vi "Generate Sine SweepV4.vi"() -> ()   [LabVIEW 2018]
uses:
  <vilib>/addons/_NISVFA/_Shared subVIs/Controls/svc_Channel Info.ctl
  <vilib>/addons/_NISVFA/_Shared subVIs/Controls/svc_Engineering Units Text Ring.ctl
  <vilib>/addons/_NISVFA/_Shared subVIs/Controls/svc_Weighting Filter Text Ring.ctl
  <vilib>/sound2/lvsound2.llb/Sound Output Task ID.ctl
  <vilib>/sound2/lvsound2.llb/Sound Input Task ID.ctl
  <vilib>/sound2/lvsound2.llb/Sound Data Format.ctl
  <vilib>/sound2/lvsound2.llb/Sampling Mode.ctl
  <vilib>/addons/Sound and Vibration/svt_Calibration/SVL Scale Voltage to EU (1 Ch).vi
  <vilib>/addons/_NISVFA/_Shared subVIs/Common/svc_Set SV Channel Info.vi
  <vilib>/addons/_NISVFA/_Shared subVIs/Common/svc_Set SV Channel Info (variant).vi
  <vilib>/addons/_NISVFA/_Shared subVIs/Common/SVL Set dB Reference (variant).vi
  <vilib>/sound2/lvsound2.llb/Sound Output Set Volume (Single).vi
  <vilib>/sound2/lvsound2.llb/Sound Output Write (DBL Single).vi
  <vilib>/sound2/lvsound2.llb/Sound Input Read (DBL).vi
  <vilib>/sound2/lvsound2.llb/Sound File Write Open.vi
  <vilib>/sound2/lvsound2.llb/Sound File Write (DBL Single).vi
  <vilib>/addons/_NISVFA/_Shared subVIs/Common/svc_Engineering Units to Unit Label.vi
  <vilib>/addons/_NISVFA/_Shared subVIs/Common/svc_Compute Scale Factor to Convert V to EU.vi
  <vilib>/addons/_NISVFA/_Shared subVIs/Common/svc_Compute Scale Factor to Convert C to EU.vi
  <vilib>/addons/_NISVFA/_Shared subVIs/Common/svc_Set dB ref if Pascal.vi
  <vilib>/addons/_NISVFA/_Shared subVIs/Common/svc_Caller VI Returned in Error Source.vi
  <vilib>/measure/maspectr.llb/FFT Spectrum (Mag-Phase) for 1 Chan.vi
  <vilib>/addons/_NISVFA/_Baseband FFT/SVFA Frequency Response (1x1) (Mag-Phase).vi
  <vilib>/measure/maspectr.llb/FFT Power Spectrum and PSD for 1 Chan.vi
  <vilib>/addons/_NISVFA/_Generation/SoundVib_Generation.lvlib
  <vilib>/addons/Sound and Vibration/svt_Calibration/SoundVib_Calibration.lvlib
  Program Files (x86)/National Instruments/LabVIEW 2018/examples/Sound and Vibration/SoundVib_Audio Examples.lvlib
  <vilib>/measure/NI_MAPro.lvlib
panel:
  out "State":string
  in  "Volume":dbl=40.0
  in  "Data Dir":path=path "C:/MTE/Utah Core Audio Test/Data"
  out "aligned signals length":i32
  out "FFT 2":cluster{"f0":dbl, "df":dbl, "magnitude":dbl[]}[](graph)
  out "FFT":cluster{"f0":dbl, "df":dbl, "magnitude":dbl[]}(graph)
  in  "averaging parameters 2":T1={"averaging mode"=enum."RMS averaging", "weighting mode"=enum."Exponential", "number of averages"=10, "linear mode"=enum."Auto restart"}
  in  "FRF mode":enum16{"H1", "H2", "H3"}(ring)
  in  "view":T2={"dB On (T)"=TRUE, "unwrap phase (F)"=FALSE, "convert to degree (T)"=TRUE}
  in  "channel info Mic":T3={"sensor sensitivity"=1000.0, "engineering units"=1, "dB reference"=1.0, "custom label"="EU", "weighting filter"=0, "pregain"=0.0} {"pregain" format="%.2f"; "weighting filter" items=["Linear", "A-weighting", "B-weighting", "C-weighting", "ITU-R 468-4", "Dolby", "CCITT", "C-message", "Wb", "Wc", "Wd", "We", "Wf", "Wh", "Wj", "Wk", "Wm", "AES17 20 kHz lowpass", "AES17 40 kHz lowpass", "AES17 20 kHz highpass", "AES17 40 kHz highpass"]; "dB reference" format="%^.1e"; "engineering units" items=["custom..."=0, "V"=1, "A"=21, "C"=30, "pC"=31, "s"=32, "-"=29, "Pa"=2, "N"=20, "g"=3, "m/s^2"=4, "m/s"=5, "m"=6, "mm/s"=12, "mm"=13, "micron/s"=14, "micron"=15, "in/s^2"=7, "in/s"=8, "in"=9, "mil/s"=10, "mil"=11, "rad/s^2"=16, "rad/s"=17, "rad"=18, "deg/s^2"=26, "deg/s"=27, "deg"=28, "RPM"=22, "cycle/s^2"=23, "Hz"=24, "cycle"=25, "strain"=19]; "sensor sensitivity" format="%#_5f"}
  in  "channel info Spk":T3={"sensor sensitivity"=1000.0, "engineering units"=1, "dB reference"=1.0, "custom label"="EU", "weighting filter"=0, "pregain"=0.0} {"pregain" format="%.2f"; "weighting filter" items=["Linear", "A-weighting", "B-weighting", "C-weighting", "ITU-R 468-4", "Dolby", "CCITT", "C-message", "Wb", "Wc", "Wd", "We", "Wf", "Wh", "Wj", "Wk", "Wm", "AES17 20 kHz lowpass", "AES17 40 kHz lowpass", "AES17 20 kHz highpass", "AES17 40 kHz highpass"]; "dB reference" format="%^.1e"; "engineering units" items=["custom..."=0, "V"=1, "A"=21, "C"=30, "pC"=31, "s"=32, "-"=29, "Pa"=2, "N"=20, "g"=3, "m/s^2"=4, "m/s"=5, "m"=6, "mm/s"=12, "mm"=13, "micron/s"=14, "micron"=15, "in/s^2"=7, "in/s"=8, "in"=9, "mil/s"=10, "mil"=11, "rad/s^2"=16, "rad/s"=17, "rad"=18, "deg/s^2"=26, "deg/s"=27, "deg"=28, "RPM"=22, "cycle/s^2"=23, "Hz"=24, "cycle"=25, "strain"=19]; "sensor sensitivity" format="%#_5f"}
  out "error out 2":errorcluster
  out "FRF":cluster{"f0":dbl, "df":dbl, "magnitude":dbl[]}(graph)
  out "Waveform Mic":waveform(dbl)[](graph)
  in  "error in (no error)":errorcluster
  in  "Samples/Sec":dbl=44100.0
  in  "Amplitude":dbl(slide)=1.0 min=0.0 max=1.0 scale=0.0..1.0
  in  "device In":u32
  out "Dur(s)":dbl
  out "error out":errorcluster
  in  "device Out":u32=1
  in  "Duration[s]":dbl=1.0
  in  "Freq Spacing":enum16{"Linear", "Logarithmic"}(ring)=enum."Logarithmic"
  out "Waveform Out":waveform(dbl)(graph)
  in  "frequency range [Hz]":cluster{"start":dbl, "stop":dbl}={"start"=20.0, "stop"=20000.0} {"stop" format="%.2f"; "start" format="%.2f"}
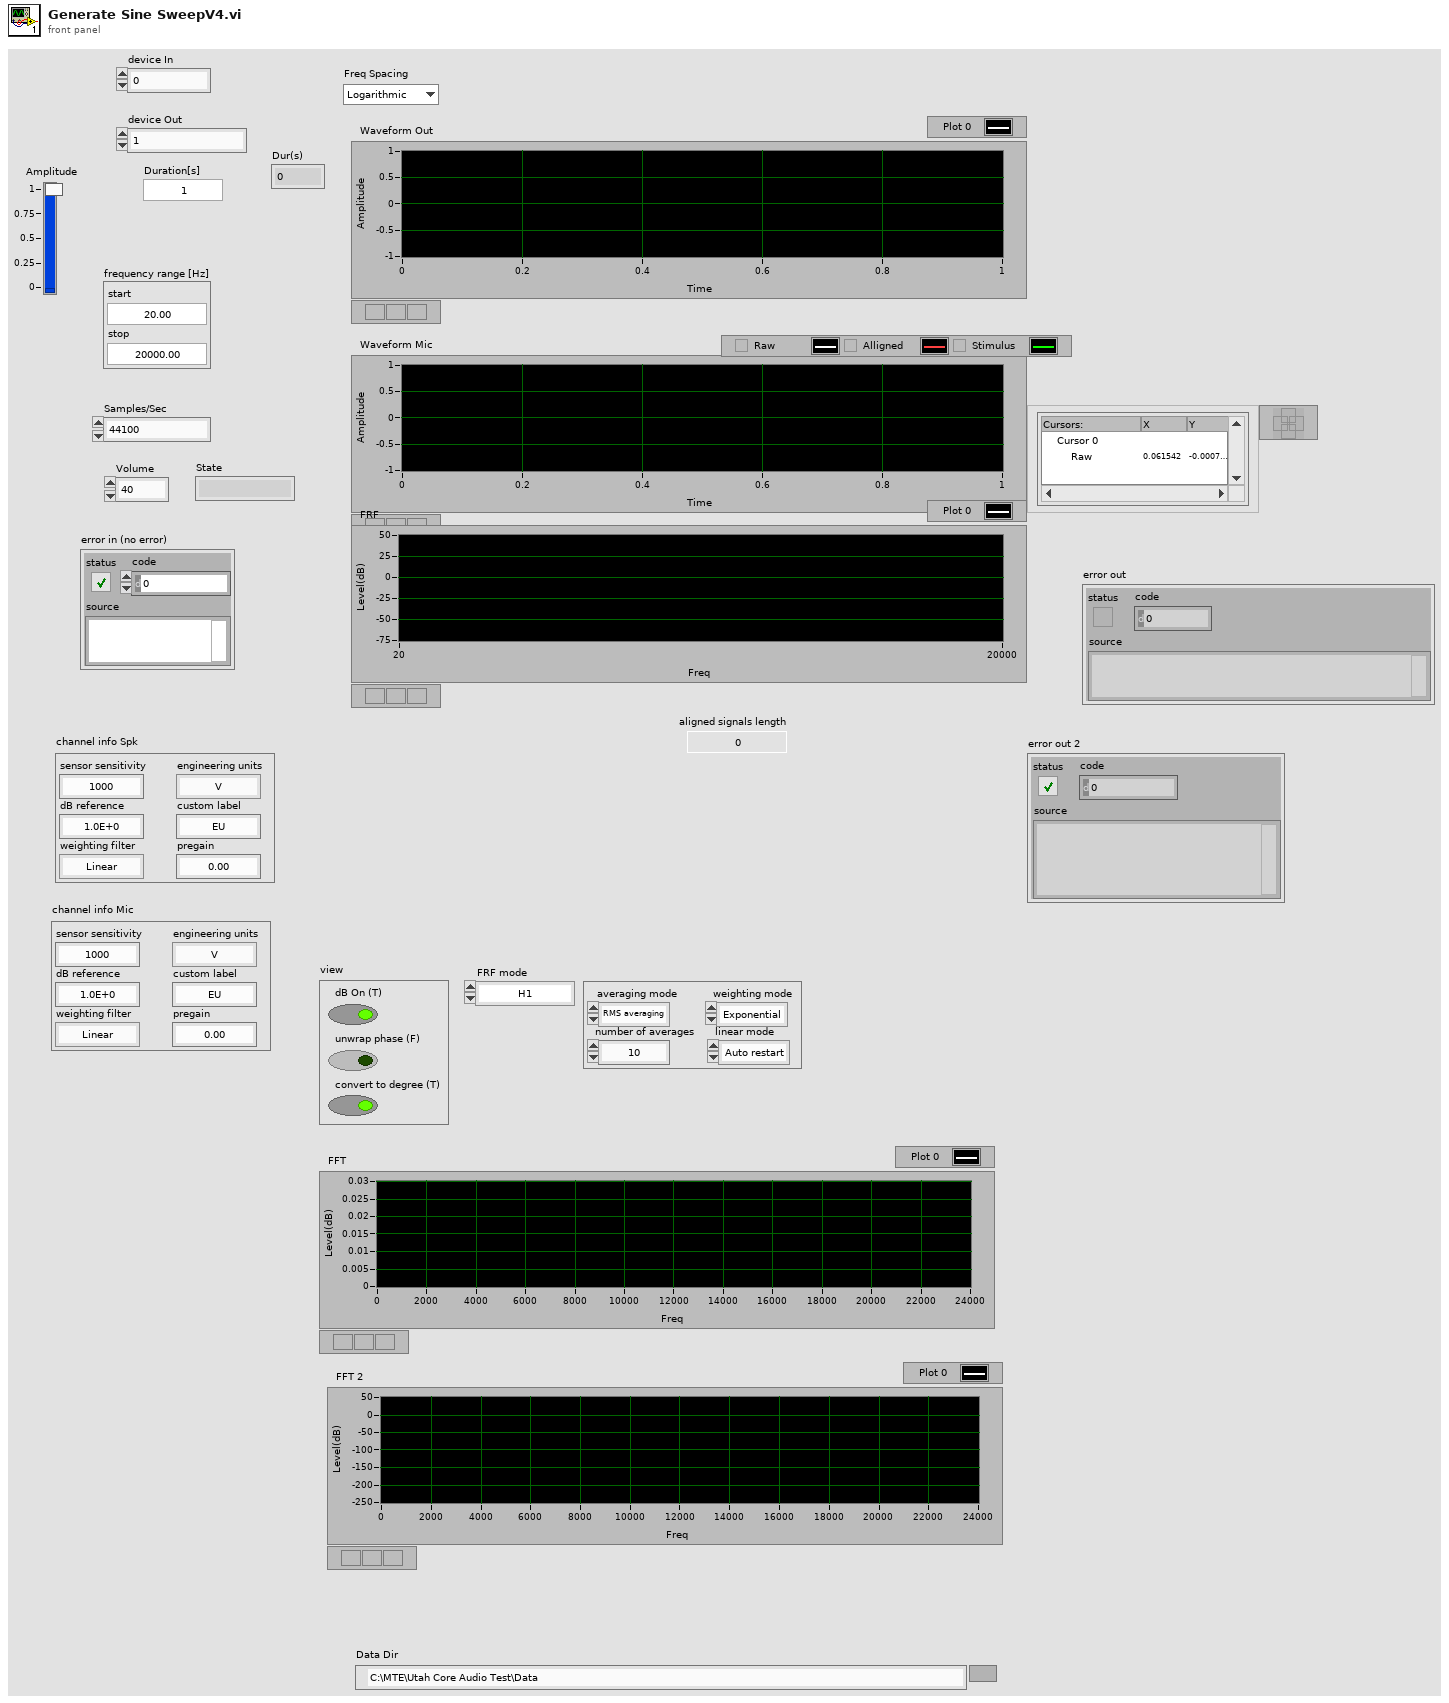
[diagram p1: front panel]
types:
  T1 = cluster{"averaging mode":enum16{"No averaging", "Vector averaging", "RMS averaging", "Peak hold"}, "weighting mode":enum16{"Linear", "Exponential"}, "number of averages":u32, "linear mode":enum16{"One shot", "Auto restart"}}
  T2 = cluster{"dB On (T)":bool, "unwrap phase (F)":bool, "convert to degree (T)":bool}
  T3 = typedef "svc_Channel Info.ctl" = cluster{"sensor sensitivity":dbl, "engineering units":T4, "dB reference":dbl, "custom label":string, "weighting filter":T5, "pregain":dbl}
  T4 = typedef "svc_Engineering Units Text Ring.ctl" = u16
  T5 = typedef "svc_Weighting Filter Text Ring.ctl" = u16
  T6 = typedef "Sound Data Format.ctl" = cluster{"sample rate (S/s)":dbl, "number of channels":i32, "bits per sample":i32}
  T7 = typedef "Sound Input Task ID.ctl" = u32
  T8 = typedef "Sound Output Task ID.ctl" = u32
  T9 = cluster{"Start":dbl, "TaskPlay":T8, "TaskMic":T7, "SampleInfo":cluster{"Fs":dbl, "#s":u32}, "Waveform":waveform(dbl), "Samples/Sec":dbl, "Duration[s]":dbl, "Mic":waveform(dbl)[], "RcdSmpl":i32, "SoundFmt":T6}
  T10 = typedef "Sampling Mode.ctl" = i32
  T11 = typedef "Sound File Refnum.ctl" = refnum<file>
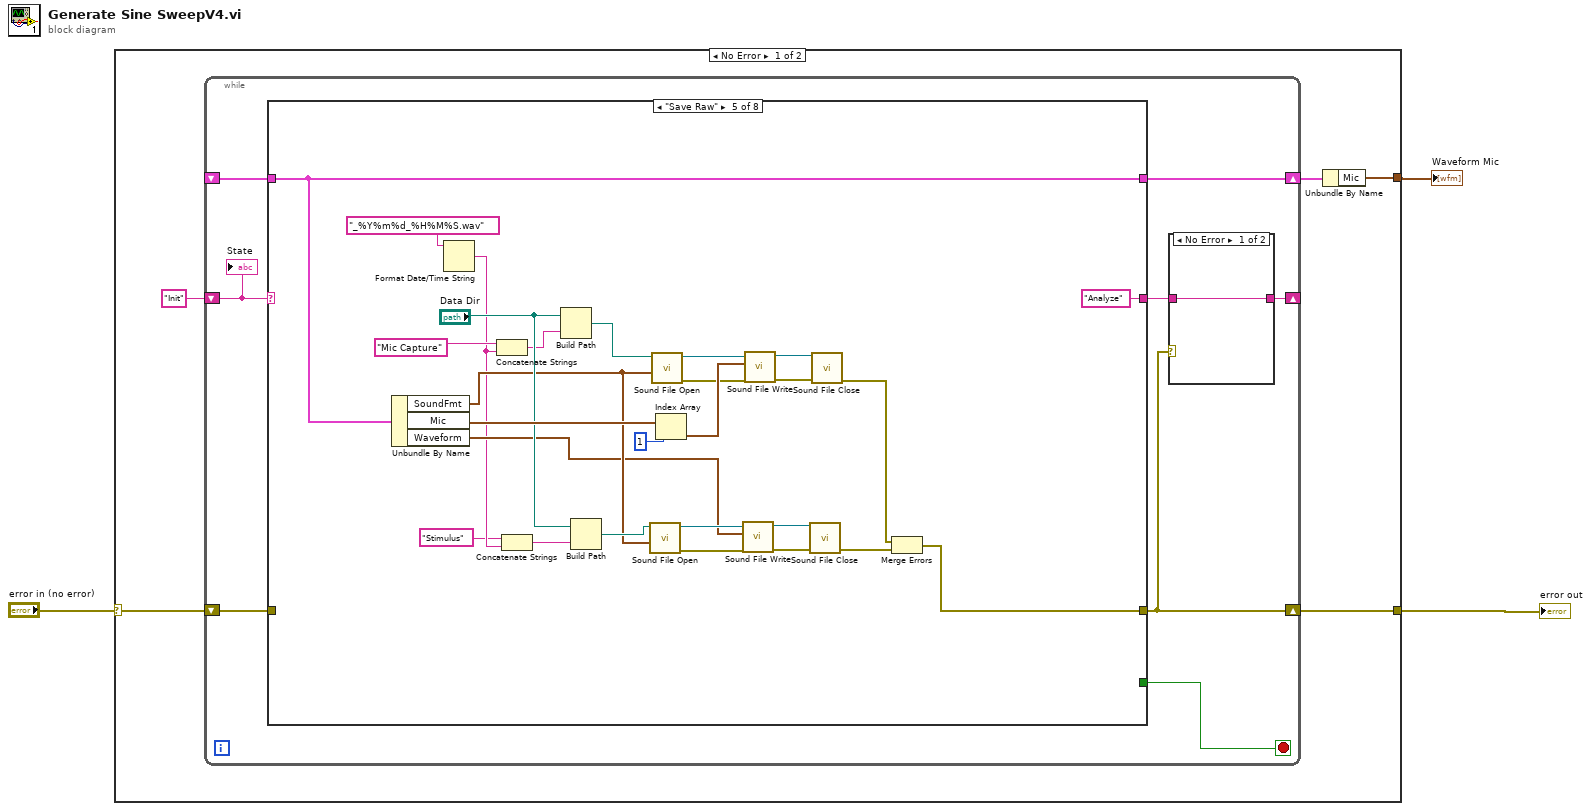
[diagram p0: block diagram]
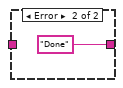
[diagram p2: hidden frame]
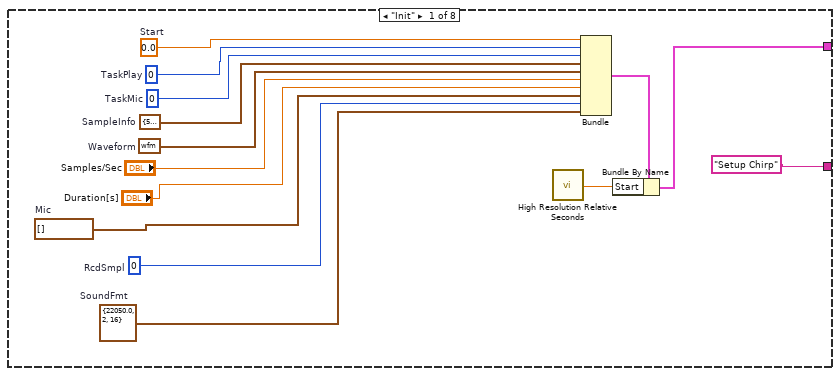
[diagram p3: hidden frame]
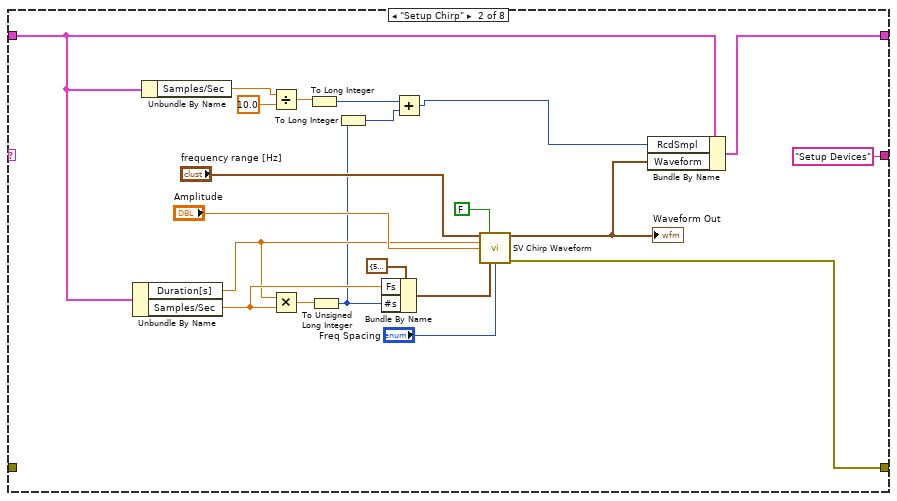
[diagram p4: hidden frame]
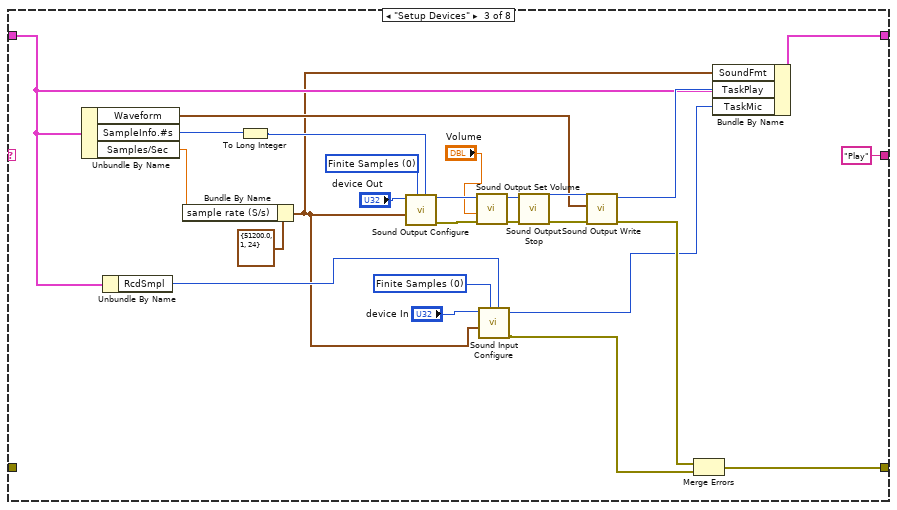
[diagram p5: hidden frame]
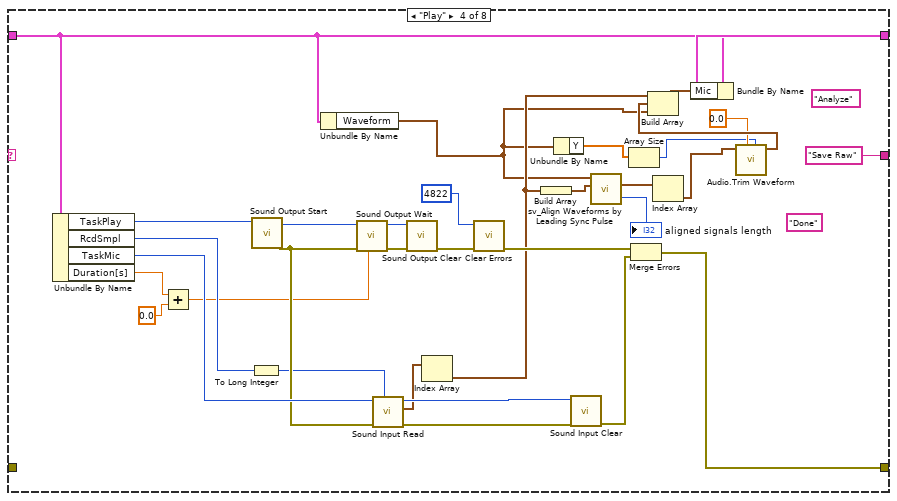
[diagram p6: hidden frame]
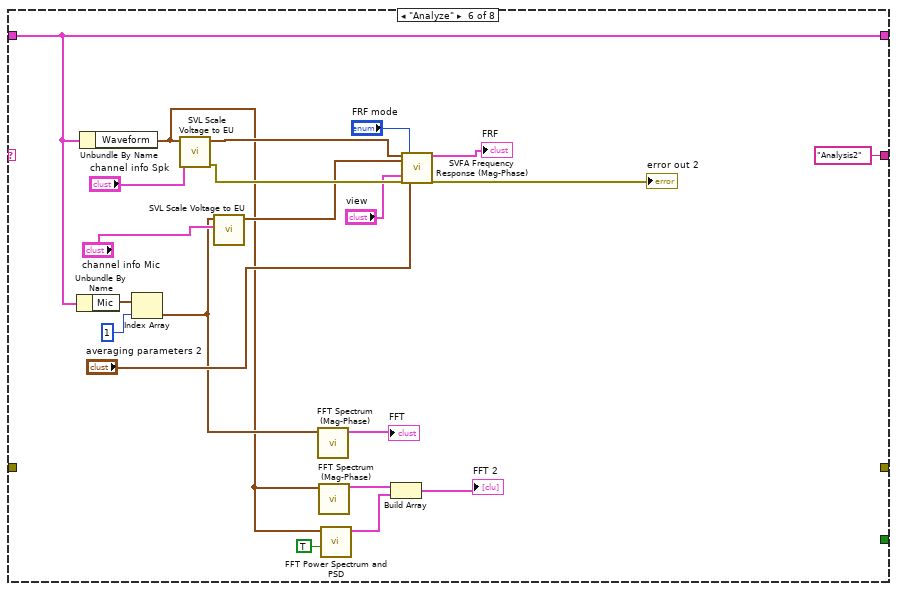
[diagram p7: hidden frame]
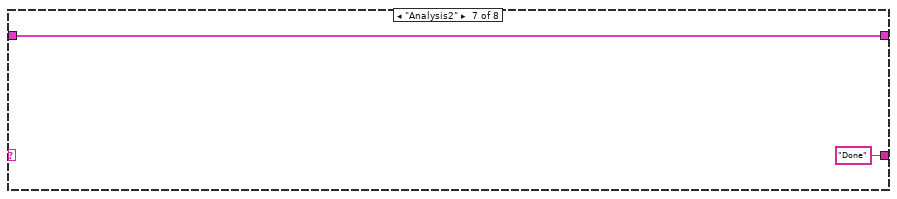
[diagram p8: hidden frame]
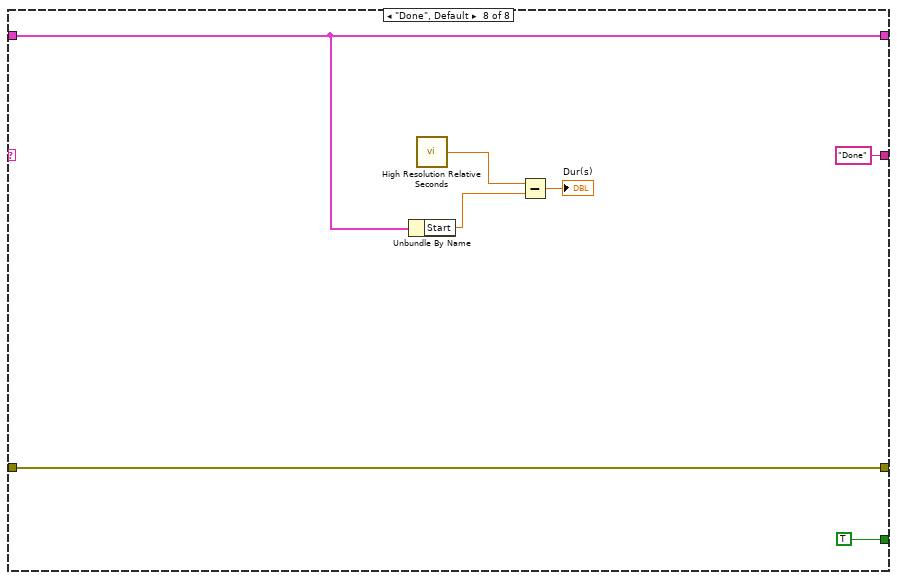
[diagram p9: hidden frame]
diagram:
  n1 = case shown="No Error" "error in (no error)" {
    selector: "error in (no error)" -> [w7 w170]
    tunnel: [w6 w170] -> w2
    tunnel: [w4 _] -> w1
    frame No Error {
      n2 = while {
        shift-right: [w12] -> _
        shift-left: "Init" -> [w16]
        shift-right: [w14] -> w5
        shift-left: _ -> [w15]
        shift-right: [w13] -> w6
        shift-left: w7 -> [w10]
        stop <- w9 stop-if-true
        n3 = case shown="\"Save Raw\"" w16 {
          tunnel: w15 -> [_ w40 w57 w91 w130 w153 w161 w165]
          tunnel: ["Setup Chirp" "Setup Devices" "Play" "Save Raw" "Analyze" "Analysis2" "Done" "Done"] -> w11
          tunnel: [w24 w45 w74 w106 w130 w153 w161 w165] -> w14
          tunnel: [_ w44 w73 w107 w119 _ _ w169] -> w13
          tunnel: w10 -> [_ _ _ _ _ _ _ w169]
          tunnel: [_ _ _ _ _ _ _ TRUE] -> w9
          frame "Init" {
            w19 = T6 {"sample rate (S/s)"=22050.0, "number of channels"=2, "bits per sample"=16}  # SoundFmt
            w20 = 0  # RcdSmpl
            w21 = waveform(dbl)[] []  # Mic
            w27 = waveform(dbl) {"t0"=timestamp(0 s since 1904-01-01), "dt"=1.0, "Y"=[]}  # Waveform
            w28 = cluster{"Fs":dbl, "#s":u32} {"Fs"=51200.0, "#s"=153600}  # SampleInfo
            w29 = T7 0  # TaskMic
            w30 = T8 0  # TaskPlay
            w31 = 0.0  # Start
            n4 = call <vilib>:"High Resolution Relative Seconds.vi"() -> ("relative seconds"=w23:dbl)
            n5 = Bundle("Start"=w31, "TaskPlay"=w30, "TaskMic"=w29, "SampleInfo"=w28, "Waveform"=w27, "Samples/Sec"="Samples/Sec", "Duration[s]"="Duration[s]", "Mic"=w21, "RcdSmpl"=w20, "SoundFmt"=w19) -> (w25:T9)  [unwired: 1 in]
            n6 = Bundle By Name(cluster=w25, "Start"=w23) -> (w24:T9)
          }
          frame "Setup Chirp" {
            n7 = Unbundle By Name(w40) -> ("Duration[s]"=w41:dbl, "Samples/Sec"=w46:dbl)
            n8 = Unbundle By Name(w40) -> ("Samples/Sec"=w39:dbl)
            n9 = Divide(x=w39, y=10.0) -> (x/y=w37:dbl)
            n10 = Multiply(x=w41, y=w46) -> (x*y=w50:dbl)
            n11 = To Long Integer(number=w37) -> (32bit integer=w36:i32)
            n12 = To Unsigned Long Integer(number=w50) -> (unsigned 32bit integer=w35:u32)
            n13 = To Long Integer(number=w35) -> (32bit integer=w33:i32)
            n14 = Bundle By Name(cluster=cluster{"Fs":dbl, "#s":u32} {"Fs"=51200.0, "#s"=153600} ("sampling info"), "Fs"=w46, "#s"=w35) -> (w53:cluster{"Fs":dbl, "#s":u32})
            n15 = Add(x=w36, y=w33) -> (x+y=w34:i32)
            n16 = call <vilib>:"SV Chirp Waveform.vi"("frequency range"="frequency range [Hz]", "reset signal (F)"=FALSE, "chirp duration [s]"=w41, "amplitude"="Amplitude", "sampling info"=w53, "frequency spacing"="Freq Spacing") -> ("chirp signal"=w42:waveform(dbl), "error out"=w44:errorcluster)  [unwired: 7 in, 1 out]
            "Waveform Out" <- w42
            n17 = Bundle By Name(cluster=w40, "RcdSmpl"=w34, "Waveform"=w42) -> (w45:T9)
          }
          frame "Setup Devices" {
            w69 = T10 0 items=["Finite Samples", "Continuous Samples"] ("sample mode")
            w76 = T10 0 items=["Finite Samples", "Continuous Samples"] ("sample mode")
            n18 = Unbundle By Name(w57) -> ("Waveform"=w62:waveform(dbl), "SampleInfo.#s"=w71:u32, "Samples/Sec"=w70:dbl)
            n19 = Unbundle By Name(w57) -> ("RcdSmpl"=w56:i32)
            n20 = Bundle By Name(cluster=T6 {"sample rate (S/s)"=51200.0, "number of channels"=1, "bits per sample"=24} ("sound format"), "sample rate (S/s)"=w70) -> (w55:T6)
            n21 = To Long Integer(number=w71) -> (32bit integer=w58:i32)
            n22 = call <vilib>:"Sound Output Configure.vi"("number of samples/ch"=w58, "sample mode"=w76, "sound format"=w55, "device ID"="device Out") -> ("error out"=w79:errorcluster, "task ID"=w78:T8)  [unwired: 6 in]
            n23 = call-poly <vilib>:"Sound Output Set Volume.vi"("error in (no error)"=w79, "volume"="Volume", "task ID"=w78) -> ("error out"=w67:errorcluster, "task ID out"=w68:T8)  [unwired: 7 in]
            n24 = call <vilib>:"Sound Input Configure.vi"("number of samples/ch"=w56, "sample mode"=w69, "sound format"=w55, "device ID"="device In") -> ("error out"=w59:errorcluster, "task ID"=w60:T7)  [unwired: 6 in]
            n25 = call <vilib>:"Sound Output Stop.vi"("error in (no error)"=w67, "task ID"=w68) -> ("error out"=w65:errorcluster, "task ID out"=w66:T8)  [unwired: 8 in]
            n26 = call-poly <vilib>:"Sound Output Write.vi"("error in (no error)"=w65, "data"=w62, "task ID"=w66) -> ("error out"=w64:errorcluster, "task ID out"=w63:T8)  [unwired: 7 in]
            n27 = Merge Errors(w64, w59) -> (w73:errorcluster)
            n28 = Bundle By Name(cluster=w57, "SoundFmt"=w55, "TaskPlay"=w63, "TaskMic"=w60) -> (w74:T9)
          }
          frame "Play" {
            (unwired) "Analyze"
            (unwired) "Done"
            n29 = Unbundle By Name(w91) -> ("TaskPlay"=w105:T8, "RcdSmpl"=w100:i32, "TaskMic"=w102:T7, "Duration[s]"=w97:dbl)
            n30 = Add(x=w97, y=0.0) -> (x+y=w95:dbl)
            n31 = To Long Integer(number=w100) -> (32bit integer=w86:i32)
            n32 = call <vilib>:"Sound Output Start.vi"("task ID"=w105) -> ("error out"=w101:errorcluster, "task ID out"=w104:T8)  [unwired: 9 in]
            n33 = Unbundle By Name(w91) -> ("Waveform"=w82:waveform(dbl))
            n34 = call <vilib>:"Sound Output Wait.vi"("timeout (sec)"=w95, "error in (no error)"=w101, "task ID"=w104) -> ("error out"=w112:errorcluster, "task ID out"=w108:T8)  [unwired: 7 in]
            n35 = call-poly <vilib>:"Sound Input Read.vi"("number of samples/ch"=w86, "error in (no error)"=w101, "task ID"=w102) -> ("error out"=w111:errorcluster, "data"=w98:waveform(dbl)[], "task ID out"=w110:T7)  [unwired: 6 in]
            n36 = call <vilib>:"Sound Output Clear.vi"("error in (no error)"=w112, "task ID"=w108) -> ("error out"=w94:errorcluster)  [unwired: 9 in]
            n37 = Index Array(array=w98) -> (element=w88:waveform(dbl))  [unwired: 1 in]
            n38 = call <vilib>:"Clear Errors.vi"("error in (no error)"=w94, "specific error code to clear (0: all)"=4822) -> ("error out"=w93:errorcluster)  [unwired: 4 in, 1 out]
            n39 = Build Array(w88) -> (w90:waveform(dbl)[])
            n40 = Unbundle By Name(w82) -> ("Y"=w81:dbl[])
            n41 = call <vilib>:"Sound Input Clear.vi"("error in (no error)"=w111, "task ID"=w110) -> ("error out"=w109:errorcluster)  [unwired: 9 in]
            n42 = call "sv_Align Waveforms by Leading Sync Pulse.vi"("response signals"=w90, "alignment reference signal"=w82) -> ("aligned signals"=w89:waveform(dbl)[], "aligned signals length"=→"aligned signals length":i32)  [unwired: 5 in, 3 out]
            n43 = Array Size(array=w81) -> (size(s)=w80:i32)
            n44 = Merge Errors(w93, w109) -> (w107:errorcluster)
            n45 = Index Array(array=w89) -> (element=w85:waveform(dbl))  [unwired: 1 in]
            n46 = call "Audio.Trim Waveform.vi"("Len"=w80, "Max Delay"=0.0, "Data In"=w85) -> ("Data Out"=w84:waveform(dbl))  [unwired: 8 in]
            n47 = Build Array(w88, w84, w82) -> (w103:waveform(dbl)[])
            n48 = Bundle By Name(cluster=w91, "Mic"=w103) -> (w106:T9)
          }
          frame "Save Raw" {
            n49 = Unbundle By Name(w130) -> ("SoundFmt"=w123:T6, "Mic"=w139:waveform(dbl)[], "Waveform"=w122:waveform(dbl))
            n50 = Format Date/Time String(time format string (%c)="_%Y%m%d_%H%M%S.wav") -> (date/time string=w115:string)  [unwired: 2 in]
            n51 = Concatenate Strings("Mic Capture" ("name or relative path"), w115) -> (w116:string)
            n52 = Concatenate Strings("Stimulus" ("name or relative path"), w115) -> (w113:string)
            n53 = Build Path(base path="Data Dir", name or relative path=w116) -> (appended path=w137:path)
            n54 = Build Path(base path="Data Dir", name or relative path=w113) -> (appended path=w124:path)
            n55 = call-poly <vilib>:"Sound File Open.vi"("sound format"=w123, "path"=w124) -> ("error out"=w128:errorcluster, "sound file refnum"=w126:T11)  [unwired: 8 in]
            n56 = call-poly <vilib>:"Sound File Open.vi"("sound format"=w123, "path"=w137) -> ("error out"=w133:errorcluster, "sound file refnum"=w136:T11)  [unwired: 8 in]
            n57 = Index Array(array=w139, index=1) -> (element=w134:waveform(dbl))
            n58 = call-poly <vilib>:"Sound File Write.vi"("error in (no error)"=w128, "data"=w122, "sound file refnum"=w126) -> ("error out"=w129:errorcluster, "sound file refnum out"=w127:T11)  [unwired: 7 in]
            n59 = call-poly <vilib>:"Sound File Write.vi"("error in (no error)"=w133, "data"=w134, "sound file refnum"=w136) -> ("error out"=w132:errorcluster, "sound file refnum out"=w135:T11)  [unwired: 7 in]
            n60 = call <vilib>:"Sound File Close.vi"("error in (no error)"=w129, "sound file refnum"=w127) -> ("error out"=w121:errorcluster)  [unwired: 9 in]
            n61 = call <vilib>:"Sound File Close.vi"("error in (no error)"=w132, "sound file refnum"=w135) -> ("error out"=w120:errorcluster)  [unwired: 9 in]
            n62 = Merge Errors(w120, w121) -> (w119:errorcluster)
          }
          frame "Analyze" {
            n63 = Unbundle By Name(w153) -> ("Mic"=w159:waveform(dbl)[])
            n64 = Unbundle By Name(w153) -> ("Waveform"=w144:waveform(dbl))
            n65 = Index Array(array=w159, index=1) -> (element=w149:waveform(dbl))
            n66 = call-poly <vilib>:"SVL Scale Voltage to EU.vi"("channel info"="channel info Spk", "signal [V]"=w144) -> ("error out"=w157:errorcluster, "scaled signal [EU]"=w147:waveform(dbl))  [unwired: 7 in, 1 out]
            n67 = call-poly <vilib>:"SVL Scale Voltage to EU.vi"("channel info"="channel info Mic", "signal [V]"=w149) -> ("scaled signal [EU]"=w146:waveform(dbl))  [unwired: 7 in, 2 out]
            n68 = call-poly <vilib>:"FFT Spectrum (Mag-Phase).vi"("time signal"=w149) -> ("magnitude"=→"FFT":cluster{"f0":dbl, "df":dbl, "magnitude":dbl[]})  [unwired: 6 in, 4 out]
            n69 = call-poly <vilib>:"FFT Spectrum (Mag-Phase).vi"("time signal"=w144) -> ("magnitude"=w143:cluster{"f0":dbl, "df":dbl, "magnitude":dbl[]})  [unwired: 6 in, 4 out]
            n70 = call-poly <vilib>:"FFT Power Spectrum and PSD.vi"("dB On (F)"=TRUE, "time signal"=w144) -> ("Power Spectrum / PSD"=w142:cluster{"f0":dbl, "df":dbl, "magnitude":dbl[]})  [unwired: 6 in, 3 out]
            n71 = Build Array(w143, w142) -> (→"FFT 2":cluster{"f0":dbl, "df":dbl, "magnitude":dbl[]}[])
            n72 = call-poly <vilib>:"SVFA Frequency Response (Mag-Phase).vi"("stimulus signal X [EUx]"=w147, "response signal Y [EUy]"=w146, "view"="view", "error in (no error)"=w157, "FRF mode"="FRF mode", "averaging parameters"="averaging parameters 2") -> ("magnitude [dB EUy/EUx]"=→"FRF":cluster{"f0":dbl, "df":dbl, "magnitude":dbl[]}, "error out"=→"error out 2":errorcluster)  [unwired: 5 in, 7 out]
          }
          frame "Analysis2" {
          }
          frame "Done", Default {
            n73 = Unbundle By Name(w165) -> ("Start"=w164:dbl)
            n74 = call <vilib>:"High Resolution Relative Seconds.vi"() -> ("relative seconds"=w166:dbl)
            n75 = Subtract(x=w166, y=w164) -> (x-y=→"Dur(s)":dbl)
          }
        }
        n76 = case shown="No Error" w13 {
          tunnel: [w17 "Done"] -> w12
          tunnel: w11 -> [w17 _]
          frame No Error {
          }
          frame Error {
          }
        }
        "State" <- w16
      }
      n77 = Unbundle By Name(w5) -> ("Mic"=w4:waveform(dbl)[])
    }
    frame Error {
    }
  }
  "error out" <- w2
  "Waveform Mic" <- w1
